vi "KE_scan_time_calc.vi"(6 "Nr. of Steps":u32=10, 8 "Start time":timestamp, 9 "wait time (ms)":u32=100, 10 "Integration Time per Step (ms)":u32=1500, 11 "move time (ms)":u32) -> (0 "Estimated stop time":timestamp, 5 "Scan Time":dbl, 7 "Start time out":timestamp)   [LabVIEW 2018]
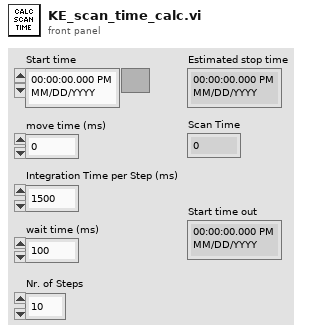
[diagram p1: front panel]
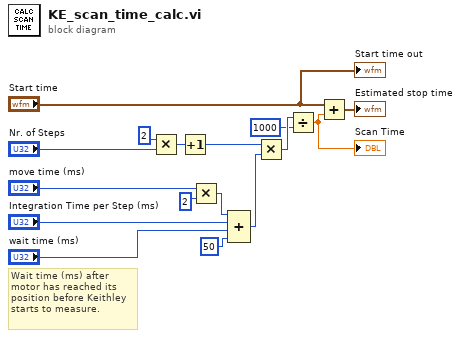
[diagram p0: block diagram]
diagram:
  # "Wait time (ms) after\nmotor has reached its\nposition before Keithley\nstarts to measure."
  n1 = Multiply(x=u32 2 ("y"), y="Nr. of Steps") -> (x*y=w5:u32)
  n2 = Increment(x=w5) -> (x+1=w3:u32)
  n3 = Multiply(x="move time (ms)", y=u32 2) -> (x*y=w14:u32)
  n4 = Compound Arithmetic op=ADD(w14, "Integration Time per Step (ms)", "wait time (ms)", u32 50 ("value")) -> (w11:u32)
  n5 = Multiply(x=w3, y=w11) -> (x*y=w10:u32)
  n6 = Divide(x=w10, y=u32 1000 ("value")) -> (x/y=w8:dbl)
  "Scan Time" <- w8
  n7 = Add(x="Start time", y=w8) -> (x+y=→"Estimated stop time":timestamp)
  "Start time out" <- "Start time"
